vi "Oxford clear buffer.vi"(8 "error in (no error)":errorcluster, 11 "VISA resource name":refnum<visa-resource-name>) -> (0 "error out":errorcluster, 1 "status byte":u16 format="%b", 2 "read buffer":string[](array[string]), 3 "VISA resource name out":refnum<visa-resource-name>)   [LabVIEW 2019]
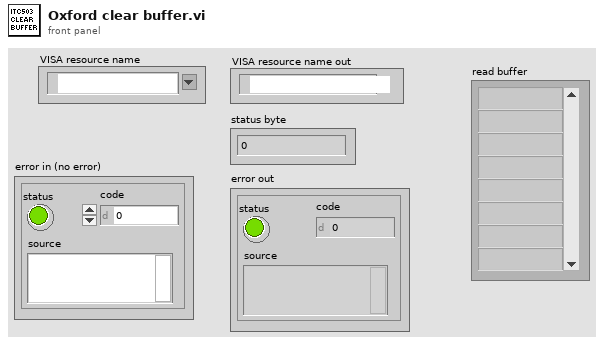
[diagram p1: front panel]
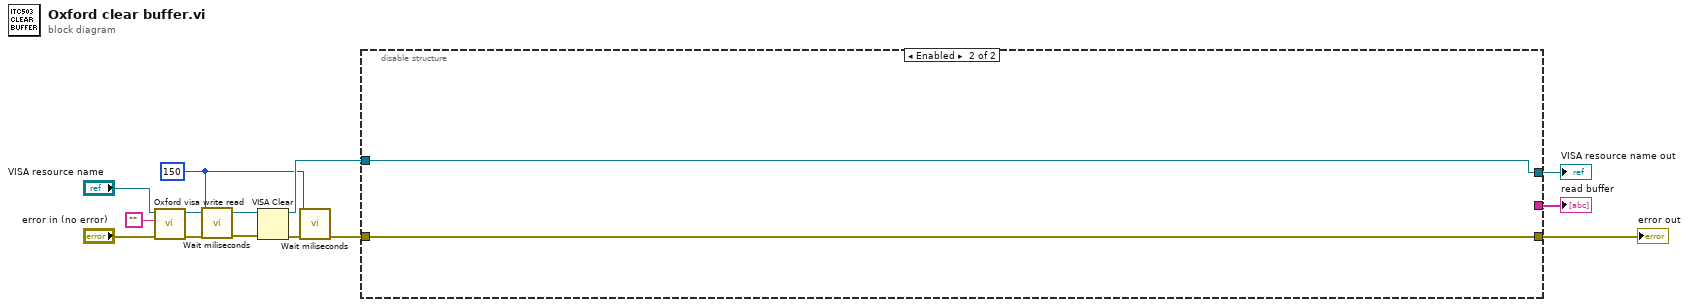
[diagram p0: block diagram]
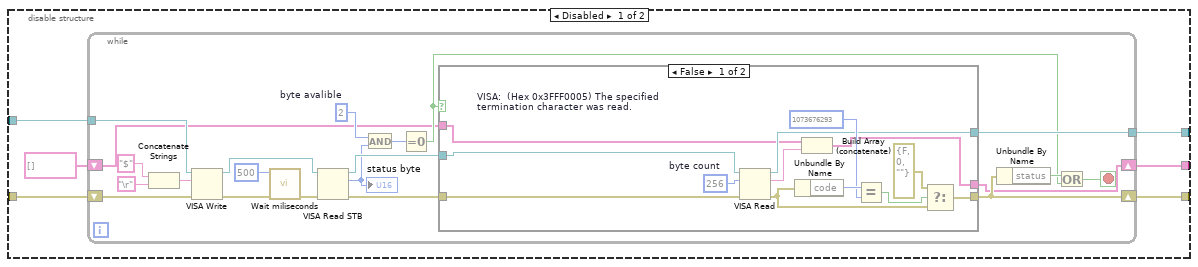
[diagram p2: hidden frame]
diagram:
  w1 = u32 150 ("milliseconds to wait")
  n1 = call "Oxford visa write read.vi"("error in (no error)"="error in (no error)", "write buffer"="", "VISA resource name"="VISA resource name") -> ("error out"=w3:errorcluster, "VISA resource name out"=w8:refnum<visa-resource-name>)  [unwired: 6 in, 1 out]
  n2 = call "Wait miliseconds.vi"("error in (no error)"=w3, "milliseconds to wait"=w1) -> ("error out"=w2:errorcluster)  [unwired: 8 in, 1 out]
  n3 = VISA Clear(VISA resource name=w8, error in (no error)=w2) -> (VISA resource name out=w7:refnum<visa-resource-name>, error out=w6:errorcluster)
  n4 = call "Wait miliseconds.vi"("error in (no error)"=w6, "milliseconds to wait"=w1) -> ("error out"=w5:errorcluster)  [unwired: 8 in, 1 out]
  n5 = disable-structure shown="Enabled" {
    disable-tunnel: [w19 w58] -> w13
    disable-tunnel: [w18 w57] -> w12
    disable-tunnel: [w17 _] -> w10
    disable-tunnel: w7 -> [w15 w57]
    disable-tunnel: w5 -> [w14 w58]
    frame Disabled {
      n6 = while {
        tunnel: [w34] -> w18
        tunnel: w15 -> [w31]
        shift-right: [w25] -> w19
        shift-left: w14 -> [w38]
        shift-right: [w21] -> w17
        shift-left: string[] [] -> [w20]
        stop <- w22 stop-if-true
        w36 = u16 2  # byte avalible
        n7 = Concatenate Strings("$" ("string"), "\r") -> (w27:string)
        n8 = VISA Write(VISA resource name=w31, write buffer=w27, error in (no error)=w38) -> (VISA resource name out=w30:refnum<visa-resource-name>, error out=w33:errorcluster)  [unwired: 1 out]
        n9 = call "Wait miliseconds.vi"("error in (no error)"=w33, "milliseconds to wait"=u32 500) -> ("error out"=w29:errorcluster)  [unwired: 8 in, 1 out]
        n10 = VISA Read STB(8:w29, 11:w30) -> (0:w40:errorcluster, 2:w37:u16, 3:w39:refnum<visa-resource-name>)
        "status byte" <- w37
        n11 = And(x=w36, y=w37) -> (x .and. y?=w35:u16)
        n12 = Equal To 0?(x=w35) -> (x = 0?=w23:bool)
        n13 = case shown="False" w23 {
          tunnel: w40 -> [w47 w56]
          tunnel: w39 -> [w46 w55]
          tunnel: [w45 w56] -> w25
          tunnel: [w44 w55] -> w34
          tunnel: [w42 w54] -> w21
          tunnel: w20 -> [w41 w54]
          frame False {
            w51 = 1073676293  # VISA:  (Hex 0x3FFF0005) The specified termination character was read.
            w53 = u32 256  # byte count
            n14 = VISA Read(VISA resource name=w46, byte count=w53, error in (no error)=w47) -> (VISA resource name out=w44:refnum<visa-resource-name>, read buffer=w43:string, error out=w50:errorcluster)  [unwired: 1 out]
            n15 = Unbundle By Name(w50) -> ("code"=w52:i32)
            n16 = Build Array (concatenate)(w41, w43) -> (w42:string[])
            n17 = Equal?(x=w52, y=w51) -> (x = y?=w49:bool)
            n18 = Select(t=errorcluster {"status"=FALSE, "code"=0, "source"=""}, s=w49, f=w50) -> (s? t:f=w45:errorcluster)
          }
          frame True {
          }
        }
        n19 = Unbundle By Name(w25) -> ("status"=w24:bool)
        n20 = Or(x=w24, y=w23) -> (x .or. y?=w22:bool)
      }
    }
    frame Enabled {
    }
  }
  "error out" <- w13
  "VISA resource name out" <- w12
  "read buffer" <- w10
